vi "auto datalogger.vi"(9 "data log interval (s)":u32=1 min=1, 11 "Datalog directory path":path) -> (0 "File Failure":bool, 3 "File refnum":refnum<file>)   [LabVIEW 2012]
uses:
  DAQ configuration/Sensor buffer command.ctl
  logic buffer cmd.ctl
  calibration/global scale array.vi
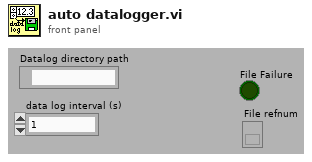
[diagram p1: front panel]
types:
  T1 = typedef "logic buffer cmd.ctl" = enum16{"read", "write ouput settings", "write rules", "write setpoints", "write output descriptions", "write all", "calculate setpoints", "save", "open", "Load all setpoint code", "Load one setpoint code", "Configure one setpoint code"}
  T2 = typedef "Sensor buffer command.ctl" = enum16{"read average", "read recent", "read all", "write", "configure", "clear"}
  T3 = enum16{"open", "open or create", "create or replace", "create", "open (read only)"}
  T4 = typedef "Sensor data.ctl" = cluster{" Sensor array":T5[], "Time":dbl}
  T5 = typedef "sensor cluster.ctl" = cluster{"voltage":sgl, "scaled":sgl, "units":string, "Out of Range":bool}
  T6 = typedef "variable setpoint.ctl" = cluster{"name":string, "unit":string, "value":dbl, "Type":enum16{"Constant", "Variable"}, "variable":cluster{"selected sensors":i32[], "selected set points":i32[], "VI":path, "Data average interval":T7, "code ref":T8}}
  T7 = typedef "data ave interval.ctl" = dbl
  T8 = typedef "type specifier for control code.ctl" = refnum<vi>
  T9 = typedef "calib array.ctl" = T10[]
  T10 = typedef "conversion.ctl" = cluster{"conversion matrix":sgl[][], "units":string, "name":string, "scale type":T11, "offset (volts)":dbl, "second channel":i8, "correspondence table":T12, "offset (physical units)":dbl, "pH scale":T13, "D.O.":T14}
  T11 = typedef "scale type.ctl" = enum16{"Volts", "Polynomial", "Correspondence Table", "pH", "Dissolved Oxygen", "Quadratic"}
  T12 = typedef "correspondence table.ctl" = cluster{"physical units":dbl, "volts":dbl}[]
  T13 = typedef "pH scale.ctl" = cluster{"Buffers":cluster{"Buffer":dbl, "Calibrated":bool, "V/T":dbl}[], "Temperature":dbl}
  T14 = typedef "DO scale.ctl" = cluster{"Temperature":dbl, "K":dbl, "barometric pressure":dbl}
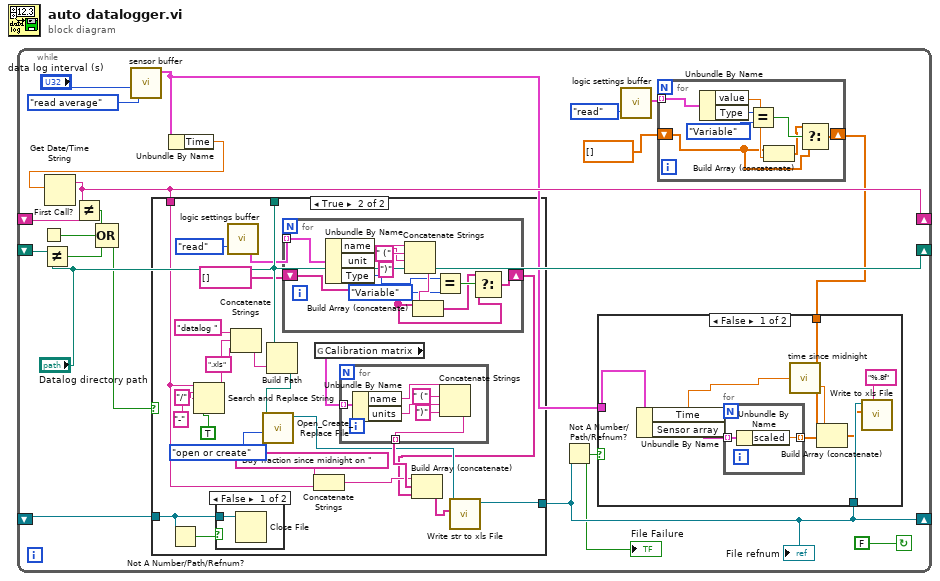
[diagram p0: block diagram]
diagram:
  n1 = while {
    shift-left: _ -> [w20]
    shift-right: ["Datalog directory path"] -> _
    shift-right: [w10] -> _
    shift-left: _ -> [w18]
    shift-right: [w13] -> _
    shift-left: _ -> [w12]
    stop <- FALSE continue-if-true
    n2 = First Call?() -> (First Call?: T/F=w16:bool)
    n3 = Not Equal?(x=w20, y="Datalog directory path") -> (x != y?=w15:bool)
    n4 = call "sensor buffer.vi"("command"=Sensor_buffer_command."read average", "smooth interval (s)"="data log interval (s)") -> ("Sensor Data smoothed"=w3:T4)  [unwired: 3 in, 2 out]
    n5 = Unbundle By Name(w3) -> ("Time"=w6:dbl)
    n6 = Get Date/Time String(seconds (now)=w6) -> (date string=w10:string)  [unwired: 2 in, 1 out]
    n7 = Not Equal?(x=w10, y=w18) -> (x != y?=w17:bool)
    n8 = Compound Arithmetic op=OR(w17, w16, w15) -> (w11:bool)
    n9 = case shown="True" w11 {
      tunnel: w12 -> [w29 w37]
      tunnel: [w29 w53] -> w13
      tunnel: "Datalog directory path" -> [_ w48]
      tunnel: w10 -> [_ w38]
      frame False {
      }
      frame True {
        n10 = Not A Number/Path/Refnum?(number/path/refnum=w37) -> (NaN/Path/Refnum?=w36:bool)
        n11 = Search and Replace String(replace all?=TRUE ("replace all? (F)"), input string=w38, search string="/", replace string="-" ("replace string (\"\")")) -> (result string=w45:string)  [unwired: 4 in, 3 out]
        n12 = case shown="False" w36 {
          tunnel: w37 -> [w66 _]
          frame False {
            n13 = Close File(refnum=w66) -> ()  [unwired: 1 in, 2 out]
          }
          frame True {
          }
        }
        n14 = call "logic settings buffer.vi"("command"=logic_buffer_cmd."read") -> ("Set Points out"=w35:T6[])  [unwired: 11 in, 7 out]
        n15 = Concatenate Strings("datalog " ("string"), w45, ".xls" ("string")) -> (w44:string)
        n16 = Build Path(base path=w48, name or relative path=w44) -> (appended path=w43:path)
        n17 = call <vilib>:"Open_Create_Replace File.vi"("function (open:0)"=T3."open or create", "file path"=w43) -> ("refnum"=w41:refnum<file>)  [unwired: 6 in, 3 out]
        n18 = for {
          tunnel: w35 -> [w65] mode=indexing
          shift-right: [w54] -> w32
          shift-left: string[] [] -> [w55]
          n19 = Unbundle By Name(w65) -> ("name"=w62:string, "unit"=w61:string, "Type"=w58:enum16{"Constant", "Variable"})
          n20 = Concatenate Strings(w62, " (" ("Substring"), w61, ")" ("Substring")) -> (w59:string)
          n21 = Build Array (concatenate)(w55, w59) -> (w56:string[])
          n22 = Equal?(x=w58, y=enum16{"Constant", "Variable"}."Variable") -> (x = y?=w60:bool)
          n23 = Select(t=w56, s=w60, f=w55) -> (s? t:f=w54:string[])
        }
        n24 = Concatenate Strings("Day fraction since midnight on " ("Substring"), w38) -> (w40:string)
        n25 = global read "global scale array.vi" "Calibration matrix"() -> (w52:T9)
        n26 = for {
          tunnel: w52 -> [w72] mode=indexing
          tunnel: [w67] -> w51 mode=indexing
          n27 = Unbundle By Name(w72) -> ("name"=w71:string, "units"=w69:string)
          n28 = Concatenate Strings(w71, " (" ("Substring"), w69, ")" ("Substring")) -> (w67:string)
        }
        n29 = Build Array (concatenate)(w40, w51, w32) -> (w31:string[])
        n30 = call "Write str to xls File.vi"("1D data"=w31, "refnum"=w41) -> ("dup refnum"=w53:refnum<file>)  [unwired: 8 in, 1 out]
      }
    }
    "File refnum" <- w13
    n31 = Not A Number/Path/Refnum?(number/path/refnum=w13) -> (NaN/Path/Refnum?=w9:bool)
    "File Failure" <- w9
    n32 = call "logic settings buffer.vi"("command"=logic_buffer_cmd."read") -> ("Set Points out"=w4:T6[])  [unwired: 11 in, 7 out]
    n33 = for {
      tunnel: w4 -> [w28] mode=indexing
      shift-right: [w22] -> w1
      shift-left: dbl[] [] -> [w21]
      n34 = Unbundle By Name(w28) -> ("value"=w24:dbl, "Type"=w27:enum16{"Constant", "Variable"})
      n35 = Equal?(x=w27, y=enum16{"Constant", "Variable"}."Variable") -> (x = y?=w25:bool)
      n36 = Build Array (concatenate)(w21, w24) -> (w23:dbl[])
      n37 = Select(t=w23, s=w25, f=w21) -> (s? t:f=w22:dbl[])
    }
    n38 = case shown="False" w9 {
      tunnel: w13 -> [w78 _]
      tunnel: w3 -> [w75 _]
      tunnel: w1 -> [w74 _]
      frame False {
        n39 = Unbundle By Name(w75) -> ("Time"=w77:dbl, "Sensor array"=w80:T5[])
        n40 = for {
          tunnel: w80 -> [w83] mode=indexing
          tunnel: [w82] -> w79 mode=indexing
          n41 = Unbundle By Name(w83) -> ("scaled"=w82:sgl)
        }
        n42 = call "time since midnight.vi"("seconds since 1Jan1904"=w77) -> ("Days"=w76:dbl)  [unwired: 1 out]
        n43 = Build Array (concatenate)(w76, w79, w74) -> (w73:dbl[])
        n44 = call "Write to xls File.vi"("format (%.3f)"="%.8f", "1D data"=w73, "refnum"=w78) -> ()  [unwired: 7 in, 2 out]
      }
      frame True {
      }
    }
  }
